vi "UDP - Datalog Sensor (SubVI).vi"(8 "error in":errorcluster, 11 "String":string="\u0002”<wy02 25\u0000\u0000\u0000mm\u0000\u0000\u0000\u0000\u0003\u0000\u0000\u0000\u0000\u0000ÈA\u0000\u0000\u0000\u0000\u000f\u0000\u0000\u0000\u0007\u0000\u0000\u0000Disp.\u0000\u0000\u0000\u0000\u0000mm\u0000\u0000\u0000\u0000\u0003p.1\u0000\u0000\u0000\u0000mm\u0000\u0000\u0001\u0000\u0000\u0000\u0002\u0000\u0000\u0000Ch3\u0000\u0000\u0000\u0000\u0000\u0000\u0000Unit\u0000\u0000\u0002\u0000\u0000\u0000\u0000\u0000\u0000\u0000\u0000\u0001\u0002\u0002\u0001\u0000\u0000\u0000\u0002\u0000\u0000\u0000Ch4\u0000\u0000\u0000\u0000\u0000\u0000\u0000Unit\u0000\u0000\u0002\u0000\u0000\u0000\u0000\u0000\u0000\u0000\u0000\u0000\u0000\u0000\u0001\u0000\u0000\u0000\u0002\u0000\u0000\u0000h") -> (0 "error out":errorcluster, 3 "Sensor Out":T1, 4 "Success":bool)   [LabVIEW 2019]
uses:
  Controls/Global - Data UDP.vi
panel:
  out "*(type *) &x":string
  out "subarray":u8[](array[numeric]) format="%.0x"
  in  "String 2":string="\u0002”<wy02 25\u0000\u0000\u0000mm\u0000\u0000\u0000\u0000\u0003\u0000\u0000\u0000\u0000\u0000ÈA\u0000\u0000\u0000\u0000\u000f\u0000\u0000\u0000\u0007\u0000\u0000\u0000Disp.\u0000\u0000\u0000\u0000\u0000mm\u0000\u0000\u0000\u0000\u0003p.1\u0000\u0000\u0000\u0000mm\u0000\u0000\u0001\u0000\u0000\u0000\u0002\u0000\u0000\u0000Ch3\u0000\u0000\u0000\u0000\u0000\u0000\u0000Unit\u0000\u0000\u0002\u0000\u0000\u0000\u0000\u0000\u0000\u0000\u0000\u0001\u0002\u0002\u0001\u0000\u0000\u0000\u0002\u0000\u0000\u0000Ch4\u0000\u0000\u0000\u0000\u0000\u0000\u0000Unit\u0000\u0000\u0002\u0000\u0000\u0000\u0000\u0000\u0000\u0000\u0000\u0000\u0000\u0000\u0001\u0000\u0000\u0000\u0002\u0000\u0000\u0000h"
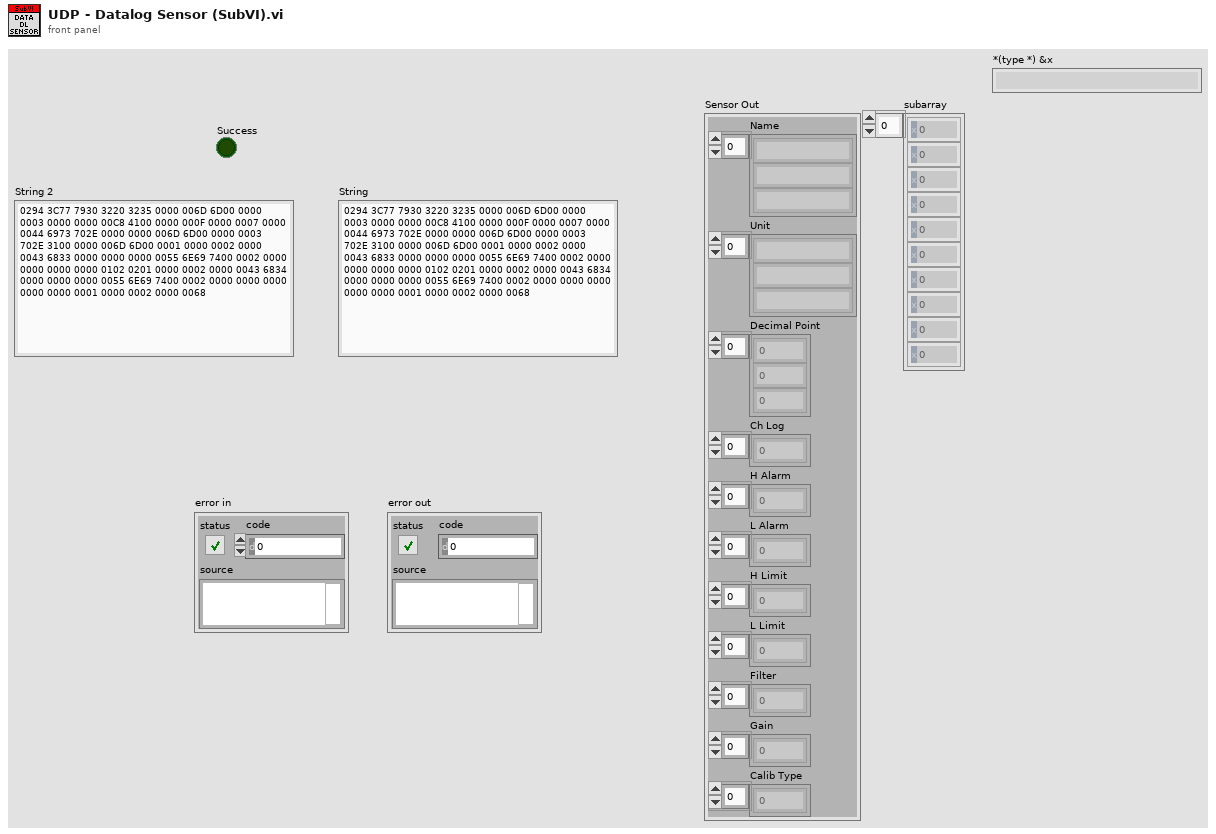
[diagram p1: front panel]
types:
  T1 = cluster{"Name":string[], "Unit":string[], "Decimal Point":u8[], "Ch Log":u8[], "H Alarm":u8[], "L Alarm":u8[], "H Limit":sgl[], "L Limit":sgl[], "Filter":u8[], "Gain":u8[], "Calib Type":u32[]}
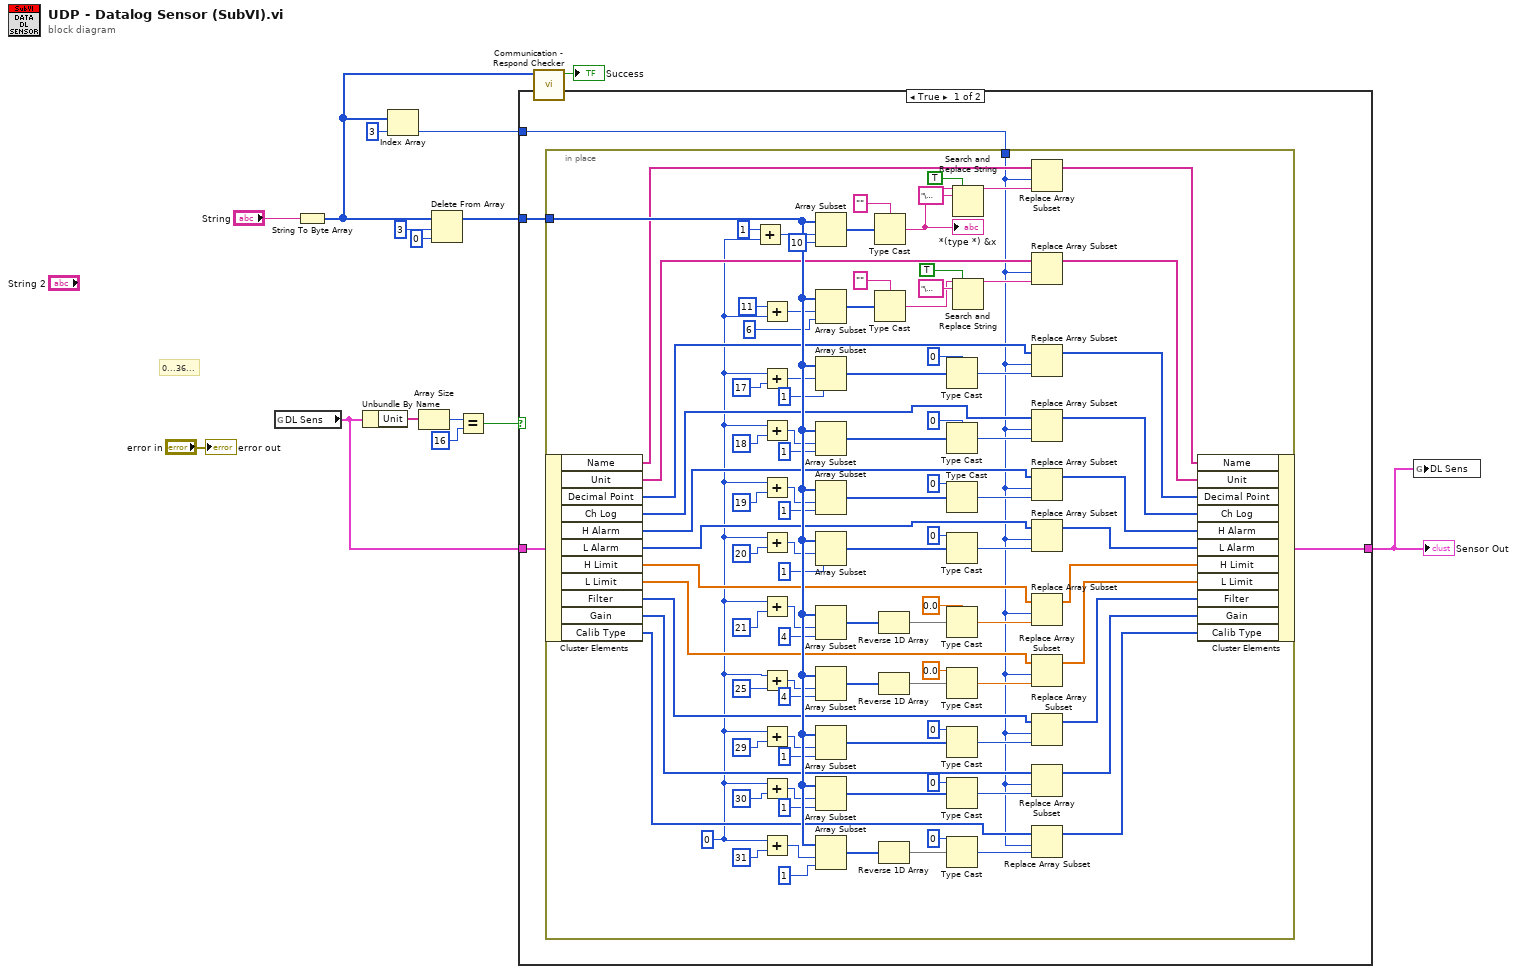
[diagram p0: block diagram]
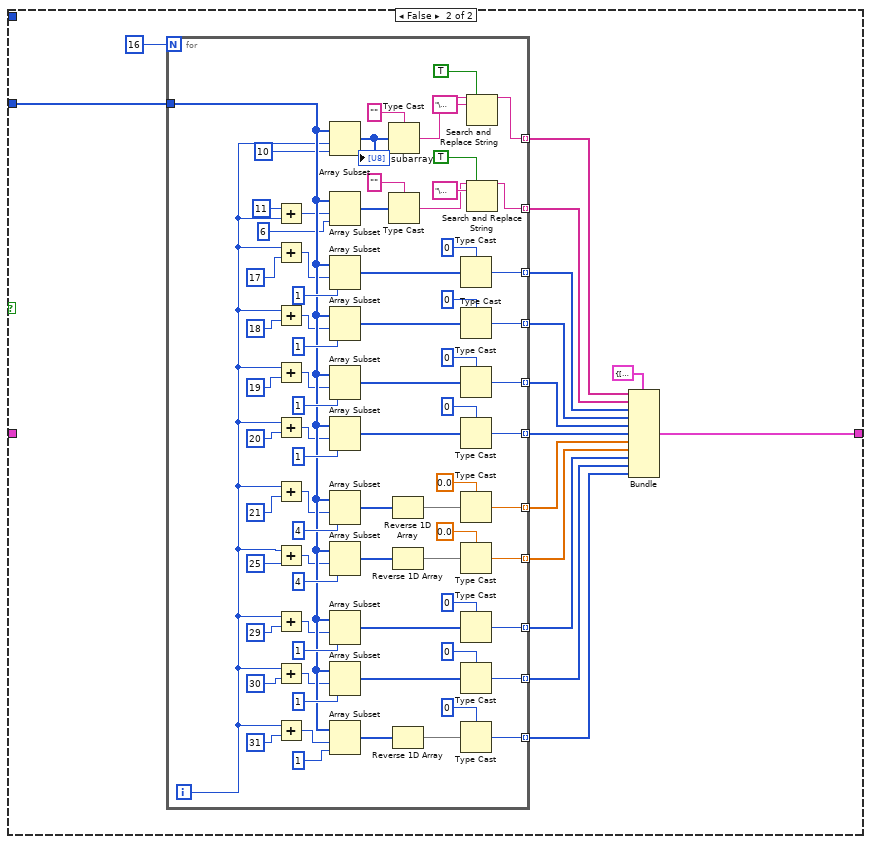
[diagram p2: hidden frame]
diagram:
  # "0...36..."
  n1 = global read "Global - Data UDP.vi" "DL Sens"() -> (w3:T1)
  n2 = String To Byte Array(string="String") -> (unsigned byte array=w9:u8[])
  n3 = Unbundle By Name(w3) -> ("Unit"=w7:string[])
  n4 = Index Array(array=w9, index=3) -> (element=w2:u8)
  n5 = Array Size(array=w7) -> (size(s)=w6:i32)
  n6 = Delete From Array(array=w9, length=3, index=0) -> (array with subset deleted=w13:u8[])  [unwired: 1 out]
  n7 = Equal?(x=w6, y=16) -> (x = y?=w4:bool)
  n8 = case shown="True" w4 {
    tunnel: w13 -> [w19 w134]
    tunnel: [w17 w120] -> w1
    tunnel: w3 -> [w18 _]
    tunnel: w2 -> [w16 _]
    frame True {
      n9 = in-place {
        in-place-border: w19 -> [w119]
        in-place-border: w16 -> [w24]
        w21 = 0
        n10 = in-place-cluster #1(w18) -> ("Name"=w56:string[], "Unit"=w54:string[], "Decimal Point"=w52:u8[], "Ch Log"=w50:u8[], "H Alarm"=w48:u8[], "L Alarm"=w46:u8[], "H Limit"=w42:sgl[], "L Limit"=w41:sgl[], "Filter"=w38:u8[], "Gain"=w37:u8[], "Calib Type"=w36:u32[])
        n11 = Add(x=1, y=w21) -> (x+y=w20:i32)
        n12 = Add(x=11, y=w21) -> (x+y=w84:i32)
        n13 = Add(x=w21, y=17 ("index")) -> (x+y=w81:i32)
        n14 = Add(x=w21, y=18 ("index")) -> (x+y=w79:i32)
        n15 = Add(x=w21, y=19 ("index")) -> (x+y=w77:i32)
        n16 = Add(x=w21, y=20 ("index")) -> (x+y=w75:i32)
        n17 = Add(x=w21, y=21 ("index")) -> (x+y=w73:i32)
        n18 = Add(x=w21, y=25 ("index")) -> (x+y=w71:i32)
        n19 = Add(x=w21, y=29 ("index")) -> (x+y=w69:i32)
        n20 = Add(x=w21, y=30 ("index")) -> (x+y=w67:i32)
        n21 = Add(x=w21, y=31 ("index")) -> (x+y=w65:i32)
        n22 = Array Subset(array=w119, index=w20, length=10) -> (w113:u8[])
        n23 = Array Subset(array=w119, index=w84, length=6) -> (w112:u8[])
        n24 = Array Subset(array=w119, index=w81, length=1) -> (w111:u8[])
        n25 = Array Subset(array=w119, index=w79, length=1) -> (w110:u8[])
        n26 = Array Subset(array=w119, index=w77, length=1) -> (w108:u8[])
        n27 = Array Subset(array=w119, index=w75, length=1) -> (w109:u8[])
        n28 = Array Subset(array=w119, index=w73, length=4) -> (w99:u8[])
        n29 = Array Subset(array=w119, index=w71, length=4) -> (w98:u8[])
        n30 = Array Subset(array=w119, index=w69, length=1) -> (w90:u8[])
        n31 = Array Subset(array=w119, index=w67, length=1) -> (w89:u8[])
        n32 = Array Subset(array=w119, index=w65, length=1) -> (w88:u8[])
        n33 = Type Cast(type="", x=w113) -> (*(type *) &x=w64:string)
        "*(type *) &x" <- w64
        n34 = Type Cast(type="", x=w112) -> (*(type *) &x=w59:string)
        n35 = Reverse 1D Array(array=w99) -> (reversed array=w97:u8[])
        n36 = Reverse 1D Array(array=w98) -> (reversed array=w96:u8[])
        n37 = Reverse 1D Array(array=w88) -> (reversed array=w87:u8[])
        n38 = Type Cast(type=u8 0, x=w111) -> (*(type *) &x=w53:u8)
        n39 = Type Cast(type=u8 0, x=w110) -> (*(type *) &x=w51:u8)
        n40 = Type Cast(type=u8 0, x=w108) -> (*(type *) &x=w49:u8)
        n41 = Type Cast(type=u8 0, x=w109) -> (*(type *) &x=w47:u8)
        n42 = Type Cast(type=sgl 0.0, x=w97) -> (*(type *) &x=w45:sgl)
        n43 = Type Cast(type=sgl 0.0, x=w96) -> (*(type *) &x=w44:sgl)
        n44 = Type Cast(type=u8 0, x=w90) -> (*(type *) &x=w43:u8)
        n45 = Type Cast(type=u8 0, x=w89) -> (*(type *) &x=w40:u8)
        n46 = Type Cast(type=u32 0, x=w87) -> (*(type *) &x=w39:u32)
        n47 = Search and Replace String(replace all?=TRUE ("replace all? (F)"), input string=w64, search string="\u0000") -> (result string=w57:string)  [unwired: 5 in, 3 out]
        n48 = Search and Replace String(replace all?=TRUE ("replace all? (F)"), input string=w59, search string="\u0000") -> (result string=w55:string)  [unwired: 5 in, 3 out]
        n49 = Replace Array Subset(array=w56, new element=w57, index=w24) -> (w35:string[])
        n50 = Replace Array Subset(array=w54, new element=w55, index=w24) -> (w34:string[])
        n51 = Replace Array Subset(array=w52, new element=w53, index=w24) -> (w33:u8[])
        n52 = Replace Array Subset(array=w50, new element=w51, index=w24) -> (w32:u8[])
        n53 = Replace Array Subset(array=w48, new element=w49, index=w24) -> (w31:u8[])
        n54 = Replace Array Subset(array=w46, new element=w47, index=w24) -> (w30:u8[])
        n55 = Replace Array Subset(array=w42, new element=w45, index=w24) -> (w29:sgl[])
        n56 = Replace Array Subset(array=w41, new element=w44, index=w24) -> (w28:sgl[])
        n57 = Replace Array Subset(array=w38, new element=w43, index=w24) -> (w27:u8[])
        n58 = Replace Array Subset(array=w37, new element=w40, index=w24) -> (w26:u8[])
        n59 = Replace Array Subset(array=w36, new element=w39, index=w24) -> (w25:u32[])
        n60 = in-place-cluster #1("Name"=w35, "Unit"=w34, "Decimal Point"=w33, "Ch Log"=w32, "H Alarm"=w31, "L Alarm"=w30, "H Limit"=w29, "L Limit"=w28, "Filter"=w27, "Gain"=w26, "Calib Type"=w25) -> (w17:T1)
      }
    }
    frame False {
      n61 = for {
        N: 16 -> [_]
        tunnel: w134 -> [w175]
        tunnel: [w153] -> w122 mode=indexing
        tunnel: [w152] -> w123 mode=indexing
        tunnel: [w151] -> w124 mode=indexing
        tunnel: [w150] -> w125 mode=indexing
        tunnel: [w149] -> w126 mode=indexing
        tunnel: [w148] -> w127 mode=indexing
        tunnel: [w147] -> w128 mode=indexing
        tunnel: [w146] -> w129 mode=indexing
        tunnel: [w145] -> w130 mode=indexing
        tunnel: [w137] -> w131 mode=indexing
        tunnel: [w143] -> w132 mode=indexing
        i -> [w135]
        n62 = Add(x=11, y=w135) -> (x+y=w173:i32)
        n63 = Add(x=w135, y=17 ("index")) -> (x+y=w170:i32)
        n64 = Add(x=w135, y=18 ("index")) -> (x+y=w168:i32)
        n65 = Add(x=w135, y=19 ("index")) -> (x+y=w166:i32)
        n66 = Add(x=w135, y=20 ("index")) -> (x+y=w164:i32)
        n67 = Add(x=w135, y=21 ("index")) -> (x+y=w162:i32)
        n68 = Add(x=w135, y=25 ("index")) -> (x+y=w160:i32)
        n69 = Add(x=w135, y=29 ("index")) -> (x+y=w158:i32)
        n70 = Add(x=w135, y=30 ("index")) -> (x+y=w156:i32)
        n71 = Add(x=w135, y=31 ("index")) -> (x+y=w154:i32)
        n72 = Array Subset(array=w175, index=w135, length=10) -> (w204:u8[])
        "subarray" <- w204
        n73 = Array Subset(array=w175, index=w173, length=6) -> (w203:u8[])
        n74 = Array Subset(array=w175, index=w170, length=1) -> (w202:u8[])
        n75 = Array Subset(array=w175, index=w168, length=1) -> (w201:u8[])
        n76 = Array Subset(array=w175, index=w166, length=1) -> (w199:u8[])
        n77 = Array Subset(array=w175, index=w164, length=1) -> (w200:u8[])
        n78 = Array Subset(array=w175, index=w162, length=4) -> (w190:u8[])
        n79 = Array Subset(array=w175, index=w160, length=4) -> (w189:u8[])
        n80 = Array Subset(array=w175, index=w158, length=1) -> (w181:u8[])
        n81 = Array Subset(array=w175, index=w156, length=1) -> (w180:u8[])
        n82 = Array Subset(array=w175, index=w154, length=1) -> (w179:u8[])
        n83 = Type Cast(type="", x=w204) -> (*(type *) &x=w144:string)
        n84 = Type Cast(type="", x=w203) -> (*(type *) &x=w138:string)
        n85 = Reverse 1D Array(array=w190) -> (reversed array=w188:u8[])
        n86 = Reverse 1D Array(array=w189) -> (reversed array=w187:u8[])
        n87 = Reverse 1D Array(array=w179) -> (reversed array=w178:u8[])
        n88 = Type Cast(type=u8 0, x=w202) -> (*(type *) &x=w145:u8)
        n89 = Type Cast(type=u8 0, x=w201) -> (*(type *) &x=w146:u8)
        n90 = Type Cast(type=u8 0, x=w199) -> (*(type *) &x=w147:u8)
        n91 = Type Cast(type=u8 0, x=w200) -> (*(type *) &x=w148:u8)
        n92 = Type Cast(type=sgl 0.0, x=w188) -> (*(type *) &x=w149:sgl)
        n93 = Type Cast(type=sgl 0.0, x=w187) -> (*(type *) &x=w150:sgl)
        n94 = Type Cast(type=u8 0, x=w181) -> (*(type *) &x=w151:u8)
        n95 = Type Cast(type=u8 0, x=w180) -> (*(type *) &x=w152:u8)
        n96 = Type Cast(type=u32 0, x=w178) -> (*(type *) &x=w153:u32)
        n97 = Search and Replace String(replace all?=TRUE ("replace all? (F)"), input string=w144, search string="\u0000") -> (result string=w143:string)  [unwired: 5 in, 3 out]
        n98 = Search and Replace String(replace all?=TRUE ("replace all? (F)"), input string=w138, search string="\u0000") -> (result string=w137:string)  [unwired: 5 in, 3 out]
      }
      n99 = Bundle(cluster=T1 {"Name"=[], "Unit"=[], "Decimal Point"=[], "Ch Log"=[], "H Alarm"=[], "L Alarm"=[], "H Limit"=[], "L Limit"=[], "Filter"=[], "Gain"=[], "Calib Type"=[]} ("output cluster"), "Name"=w132, "Unit"=w131, "Decimal Point"=w130, "Ch Log"=w129, "H Alarm"=w128, "L Alarm"=w127, "H Limit"=w126, "L Limit"=w125, "Filter"=w124, "Gain"=w123, "Calib Type"=w122) -> (w120:T1)
    }
  }
  "Sensor Out" <- w1
  n100 = call "Communication - Respond Checker.vi"("Read Data"=w9) -> ("Success"=→"Success":bool)  [unwired: 10 in]
  n101 = global write "Global - Data UDP.vi" "DL Sens"(w1) -> ()
  "error out" <- "error in"
